vi "NF90 move to position.vi"(5 "program (Run=False)":bool, 7 "Error In":errorcluster, 8 "move type (abs = False)":bool, 9 "move":T1={"axis"=enum."X", "Increment"=0.0, "Speed"=1.0, "Acceleration"=1} {"Speed" min=0 format="%.3f"; "Acceleration" min=1 max=50 step=1; "Increment" format="%.3f"}, 10 "port number in":refnum<visa-resource-name>) -> (0 "Error Out":errorcluster, 1 "killed":bool, 2 "Position out":sgl format="%.2f", 3 "port number out":refnum<visa-resource-name>)   [LabVIEW 2019]
uses:
  NF90 move.ctl
  Axis.ctl
  NF90 commands.ctl
panel:
  out "s? t:f":sgl format="%.2f"
  out "Position":sgl format="%.2f"
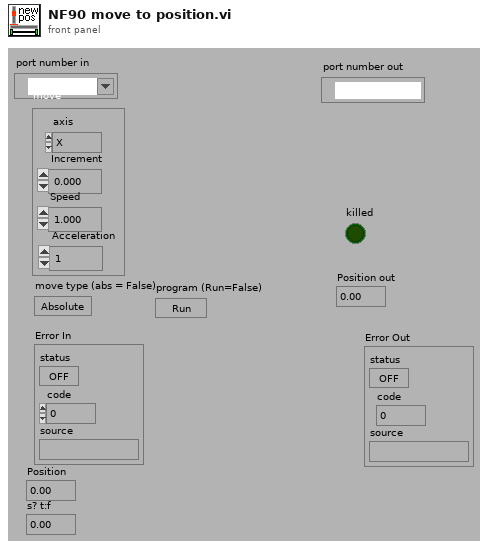
[diagram p1: front panel]
types:
  T1 = typedef "NF90 move.ctl" = cluster{"axis":T2, "Increment":sgl, "Speed":sgl, "Acceleration":u8}
  T2 = typedef "Axis.ctl" = enum16{"X", "Y", "Z"}
  T3 = typedef "NF90 commands.ctl" = enum16{"Index", "Speed", "Acceleration", "Backlash", "Quit", "Run", "Null indexes", "Verify status", "Clear program", "Computer Control", "Go", "Put Controller on Hold", "Position"}
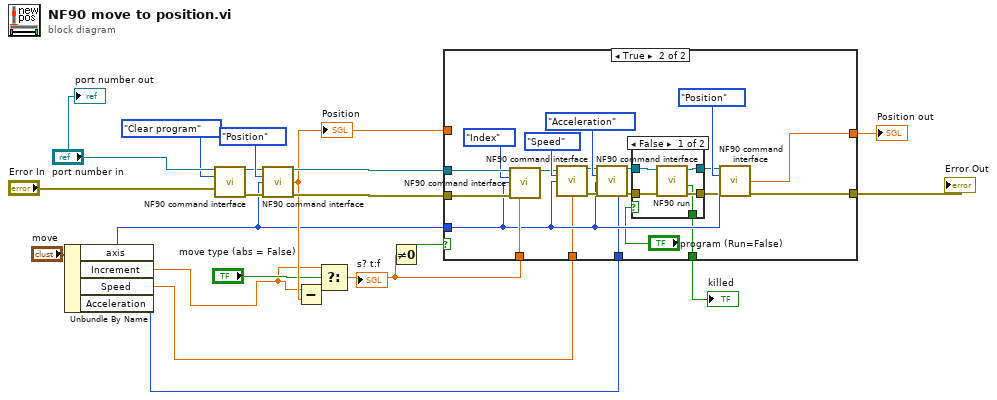
[diagram p0: block diagram]
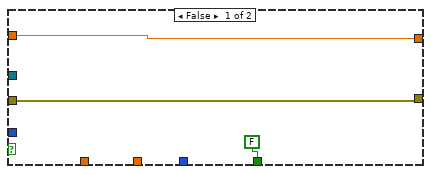
[diagram p2: hidden frame]
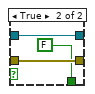
[diagram p3: hidden frame]
diagram:
  n1 = Unbundle By Name("move") -> ("axis"=w10:T2, "Increment"=w6:sgl, "Speed"=w9:sgl, "Acceleration"=w8:u8)
  n2 = call "NF90 command interface.vi"("port number in"="port number in", "commands"=NF90_commands."Clear program", "Error In"="Error In") -> ("port number out"=w17:refnum<visa-resource-name>, "Error Out"=w16:errorcluster)  [unwired: 8 in, 3 out]
  n3 = call "NF90 command interface.vi"("port number in"=w17, "commands"=NF90_commands."Position", "axis"=w10, "Error In"=w16) -> ("port number out"=w19:refnum<visa-resource-name>, "Position"=w18:sgl, "Error Out"=w20:errorcluster)  [unwired: 7 in, 2 out]
  "Position" <- w18
  n4 = Subtract(x=w6, y=w18) -> (x-y=w7:sgl)
  n5 = Select(t=w6, s="move type (abs = False)", f=w7) -> (s? t:f=w5:sgl)
  "s? t:f" <- w5
  n6 = Not Equal To 0?(x=w5) -> (x != 0?=w4:bool)
  n7 = case shown="True" w4 {
    tunnel: w20 -> [w22 w45]
    tunnel: w19 -> [_ w44]
    tunnel: w5 -> [_ w34]
    tunnel: w10 -> [_ w33]
    tunnel: w9 -> [_ w32]
    tunnel: w8 -> [_ w31]
    tunnel: [w24 w27] -> w3
    tunnel: w18 -> [w24 _]
    tunnel: [FALSE ("killed") w26] -> w2
    tunnel: [w22 w25] -> w1
    frame False {
    }
    frame True {
      n8 = call "NF90 command interface.vi"("port number in"=w44, "commands"=NF90_commands."Index", "axis"=w33, "Error In"=w45, "Distance"=w34) -> ("port number out"=w35:refnum<visa-resource-name>)  [unwired: 6 in, 4 out]
      n9 = call "NF90 command interface.vi"("port number in"=w35, "commands"=NF90_commands."Speed", "axis"=w33, "Speed"=w32) -> ("port number out"=w39:refnum<visa-resource-name>, "Error Out"=w40:errorcluster)  [unwired: 7 in, 3 out]
      n10 = call "NF90 command interface.vi"("port number in"=w39, "commands"=NF90_commands."Acceleration", "axis"=w33, "Error In"=w40, "Acceleration"=w31) -> ("port number out"=w38:refnum<visa-resource-name>, "Error Out"=w37:errorcluster)  [unwired: 6 in, 3 out]
      n11 = case shown="False" "program (Run=False)" {
        tunnel: w38 -> [w50 w53]
        tunnel: w37 -> [w49 w52]
        tunnel: [w48 w53] -> w30
        tunnel: [w47 w52] -> w29
        tunnel: [w46 FALSE ("killed")] -> w26
        frame False {
          n12 = call "NF90 run.vi"("Error In"=w49, "port number in"=w50) -> ("Error Out"=w47:errorcluster, "killed"=w46:bool, "port number out"=w48:refnum<visa-resource-name>)  [unwired: 7 in]
        }
        frame True {
        }
      }
      n13 = call "NF90 command interface.vi"("port number in"=w30, "commands"=NF90_commands."Position", "axis"=w33, "Error In"=w29) -> ("Position"=w27:sgl, "Error Out"=w25:errorcluster)  [unwired: 7 in, 3 out]
    }
  }
  "Position out" <- w3
  "killed" <- w2
  "Error Out" <- w1
  "port number out" <- "port number in"
